vi "Gen_TrajLib_Doc_TypeDef.vi"() -> ()   [LabVIEW 2019]
doc: "Generates and HTML file with the Description of every class, library, ctl, and vi in every open project. Creates separate documents for each library and virtual folder , and links to the top level document. In addition, for every VI shows connector pane. Saves the HTML file in folder <project folder>\\<project name> Documentation\\Documentation.html. erases previous content if any. \nDoes not create documentation for Documentation folder in project if exists. Does not create documentation for packed libraries in the project."
uses:
  Doc_Builder_SubVI/FileAndPath.ctl
  <vilib>/Utility/NIReport.llb/NI_report.lvclass
panel:
  out "Current Section":string
  out "File Index":i32
  out "File Count":i32
  in  "stop":bool
  out "Full Input File Name":path
  in  "GO":bool
  in  "Documentation Path":path=path "C:/Shares/Common/FRC/FRC_TrajLib/FRC_LV_Traj_Doc_Builder/Doc1/TypeDef"
  in  "Library Path":path=path "C:/Shares/github/FRC_LV_TrajLib/FRC_LV_Trajectory_Library/TypeDef"
  out "Doc Path":path
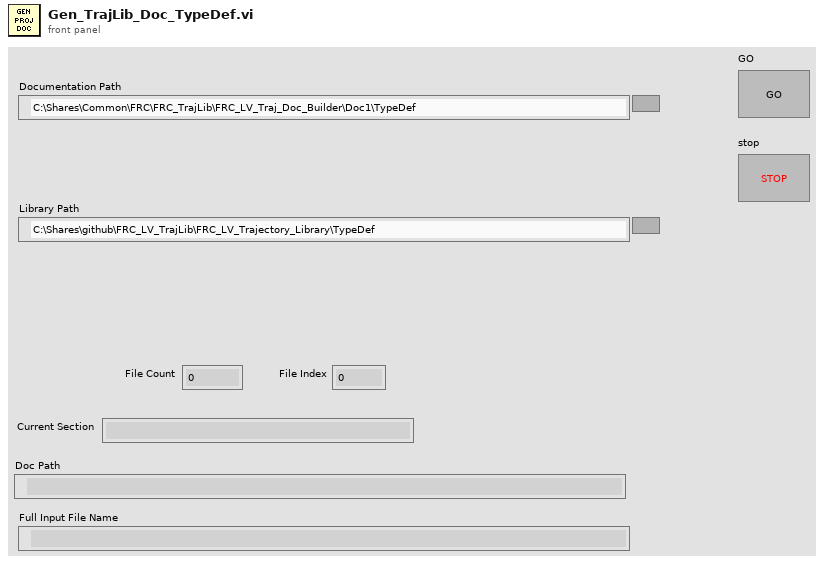
[diagram p1: front panel]
types:
  T1 = typedef "FileAndPath.ctl" = cluster{"FileName":string, "Library Path":path}
  T2 = enum16{"Standard Report", "HTML", "Word", "Excel"}
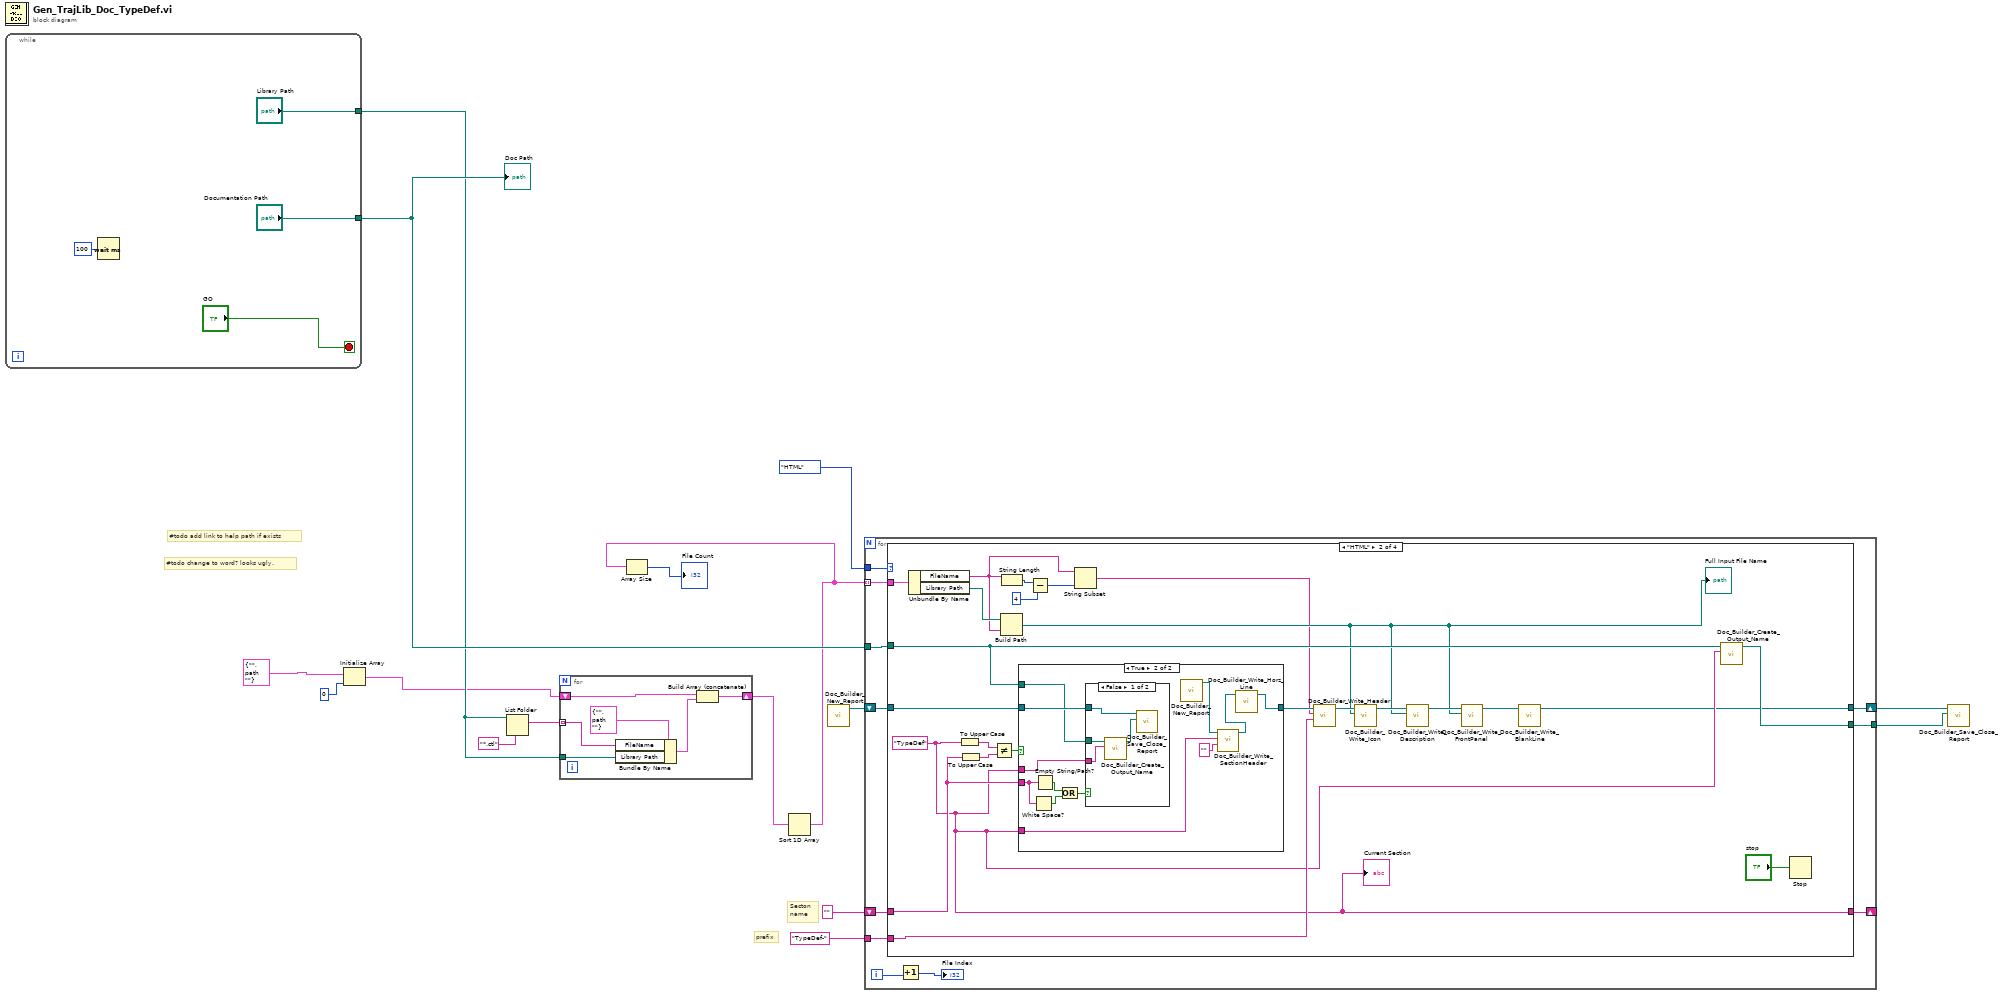
[diagram p0: block diagram]
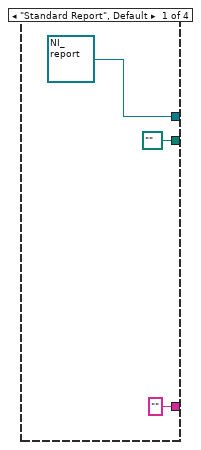
[diagram p2: hidden frame]
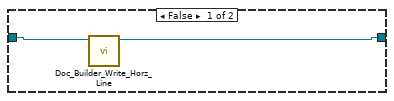
[diagram p3: hidden frame]
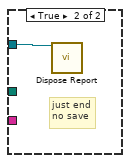
[diagram p4: hidden frame]
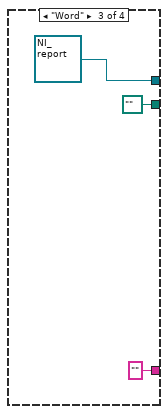
[diagram p5: hidden frame]
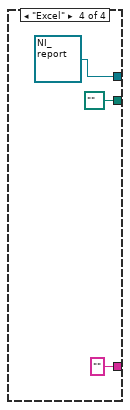
[diagram p6: hidden frame]
diagram:
  # "Secton \nname"
  # "prefix"
  # "#todo change to word? looks ugly."
  # "#todo add link to help path if exists"
  n1 = while {
    tunnel: ["Documentation Path"] -> w14
    tunnel: ["Library Path"] -> w10
    stop <- "GO" stop-if-true
    n2 = Wait (ms)(milliseconds to wait=u32 100) -> ()  [unwired: 1 out]
  }
  "Doc Path" <- w14
  n3 = Initialize Array(T1 {"FileName"="", "Library Path"=path ""} ("FileAndPath"), 0 ("dimension size")) -> (w8:T1[])
  n4 = List Folder(path=w10, pattern="*.ctl") -> (filenames=w11:string[])  [unwired: 2 in, 3 out]
  n5 = for {
    tunnel: w11 -> [w26] mode=indexing
    tunnel: w10 -> [w25]
    shift-right: [w24] -> w1
    shift-left: w8 -> [w23]
    n6 = Bundle By Name(cluster=T1 {"FileName"="", "Library Path"=path ""} ("FileAndPath"), "FileName"=w26, "Library Path"=w25) -> (w21:T1)
    n7 = Build Array (concatenate)(w23, w21) -> (w24:T1[])
  }
  n8 = Sort 1D Array(array=w1) -> (sorted array=w6:T1[])
  n9 = Array Size(array=w6) -> (size(s)=→"File Count":i32)
  n10 = call "Doc_Builder_New_Report.vi"() -> ("NI_report out"=w5:refnum<class "NI_report.lvclass">)  [unwired: 11 in]
  n11 = for {
    tunnel: w6 -> [w36] mode=indexing
    tunnel: T2."HTML" ("report type") -> [w37]
    tunnel: w14 -> [w35]
    tunnel: "TypeDef-" ("string") -> [w32]
    shift-right: [w28] -> w3
    shift-left: w5 -> [w31]
    shift-right: [w27] -> _
    shift-left: "" ("string") -> [w30]
    tunnel: [w29] -> w2
    i -> [w34]
    n12 = case shown="\"HTML\"" w37 {
      tunnel: w36 -> [_ w58 _ _]
      tunnel: w35 -> [_ w49 _ _]
      tunnel: w32 -> [_ w46 _ _]
      tunnel: w31 -> [_ w53 _ _]
      tunnel: w30 -> [_ w50 _ _]
      tunnel: [path "" ("Full Report Name") w51 path "" ("Full Report Name") path "" ("Full Report Name")] -> w29
      tunnel: [refnum<class "NI_report.lvclass"> refnum ("report out") w41 refnum<class "NI_report.lvclass"> refnum ("report out") refnum<class "NI_report.lvclass"> refnum ("report out")] -> w28
      tunnel: ["" ("FileName") w43 "" ("FileName") "" ("FileName")] -> w27
      frame "Standard Report", Default {
      }
      frame "HTML" {
        w43 = "TypeDef" ("string")
        n13 = Unbundle By Name(w58) -> ("FileName"=w56:string, "Library Path"=w57:path)
        n14 = To Upper Case(1:w43) -> (0:w55:string)
        n15 = To Upper Case(1:w50) -> (0:w54:string)
        n16 = Not Equal?(x=w55, y=w54) -> (x != y?=w44:bool)
        n17 = Build Path(base path=w57, name or relative path=w56) -> (appended path=w47:path)
        "Full Input File Name" <- w47
        n18 = String Length(string=w56) -> (length=w63:i32)
        n19 = case shown="True" w44 {
          tunnel: w53 -> [w66 w75]
          tunnel: [w65 w72] -> w52
          tunnel: w50 -> [_ w73]
          tunnel: w49 -> [_ w74]
          tunnel: w43 -> [_ w69]
          tunnel: w43 -> [_ w68]
          frame False {
            n20 = call "Doc_Builder_Write_Horz_Line.vi"("NI_report in"=w66) -> ("NI_report out"=w65:refnum<class "NI_report.lvclass">)  [unwired: 10 in]
          }
          frame True {
            n21 = White Space?(1:w73) -> (0:w77:bool)
            n22 = Empty String/Path?(string/path=w73) -> (empty?=w76:bool)
            n23 = Or(x=w76, y=w77) -> (x .or. y?=w78:bool)
            n24 = case shown="False" w78 {
              tunnel: w75 -> [w82 w83]
              tunnel: w74 -> [w81 _]
              tunnel: w68 -> [w80 _]
              frame False {
                n25 = call "Doc_Builder_Create_Output_Name.vi"("Section Name"=w80, "Path"=w81) -> ("Full Report Name"=w79:path)  [unwired: 9 in]
                n26 = call "Doc_Builder_Save_Close_Report.vi"("appended path"=w79, "NI_report in"=w82) -> ()  [unwired: 9 in, 1 out]
              }
              frame True {
                # "just end\nno save"
                n27 = call-dynamic "Dispose Report.vi"("report in"=w83) -> ()  [unwired: 14 in, 1 out]
              }
            }
            n28 = call "Doc_Builder_New_Report.vi"() -> ("NI_report out"=w71:refnum<class "NI_report.lvclass">)  [unwired: 11 in]
            n29 = call "Doc_Builder_Write_SectionHeader.vi"("Prefix String"="", "Section Name"=w69, "NI_report in"=w71) -> ("NI_report out"=w70:refnum<class "NI_report.lvclass">)  [unwired: 8 in]
            n30 = call "Doc_Builder_Write_Horz_Line.vi"("NI_report in"=w70) -> ("NI_report out"=w72:refnum<class "NI_report.lvclass">)  [unwired: 10 in]
          }
        }
        n31 = Subtract(x=w63, y=4) -> (x-y=w61:i32)
        n32 = String Subset(string=w56, length (rest)=w61) -> (substring=w45:string)  [unwired: 1 in]
        n33 = call "Doc_Builder_Write_Header.vi"("Prefix String"=w46, "Item Name"=w45, "NI_report in"=w52) -> ("NI_report out"=w60:refnum<class "NI_report.lvclass">)  [unwired: 8 in]
        n34 = call "Doc_Builder_Write_Icon.vi"("Input Item file path"=w47, "NI_report in"=w60) -> ("NI_report out"=w59:refnum<class "NI_report.lvclass">)  [unwired: 9 in]
        n35 = call "Doc_Builder_Write_Description.vi"("input item file path"=w47, "NI_report in"=w59) -> ("NI_report out"=w48:refnum<class "NI_report.lvclass">)  [unwired: 9 in]
        n36 = call "Doc_Builder_Write_FrontPanel.vi"("input item file path"=w47, "NI_report in"=w48) -> ("NI_report out"=w42:refnum<class "NI_report.lvclass">)  [unwired: 9 in]
        n37 = call "Doc_Builder_Write_BlankLine.vi"("NI_report in"=w42) -> ("NI_report out"=w41:refnum<class "NI_report.lvclass">)  [unwired: 10 in]
        n38 = call "Doc_Builder_Create_Output_Name.vi"("Section Name"=w43, "Path"=w49) -> ("Full Report Name"=w51:path)  [unwired: 9 in]
        n39 = Stop(stop? (T)="stop") -> ()
        "Current Section" <- w43
      }
      frame "Word" {
      }
      frame "Excel" {
      }
    }
    n40 = Increment(x=w34) -> (x+1=→"File Index":i32)
  }
  n41 = call "Doc_Builder_Save_Close_Report.vi"("appended path"=w2, "NI_report in"=w3) -> ()  [unwired: 9 in, 1 out]
